vi "optionsAcq_channel_PD temperature mode.vi"(6 "read/write":enum16{"read", "write"}(ring), 8 "error in (no error)":errorcluster, 10 "PD sensitivity mode write":T1, 11 "OSAchannel in":refnum<class "OSAchannel.lvclass">) -> (0 "error out":errorcluster, 1 "channel.temp Variable":bool, 2 "PD sensitivity mode out":T1, 3 "OSAchannel out":refnum<class "OSAchannel.lvclass">, 5 "status FTSLib":i32)   [LabVIEW 2010, in "OSAchannel.lvclass"]
uses:
  OSAchannel.lvclass
  _misc/Thorlabs_FTS_misc.llb/PDTemperatureMode.ctl
  OSAchannel.lvclass/OSAchannel.ctl
  _dll/LVLib/FTSLib.lvlib
  OSA20X_misc.lvlib
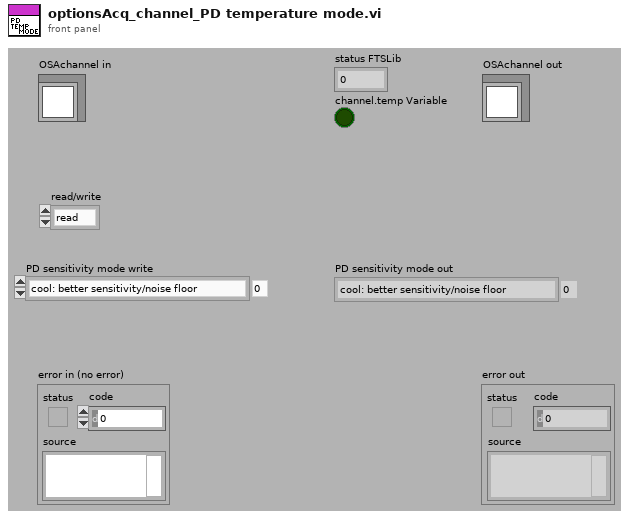
[diagram p1: front panel]
types:
  T1 = typedef "OSA20X_misc.lvlib/PDTemperatureMode.ctl" = enum16{"cool: better sensitivity/noise floor", "warm: extended wl range"}
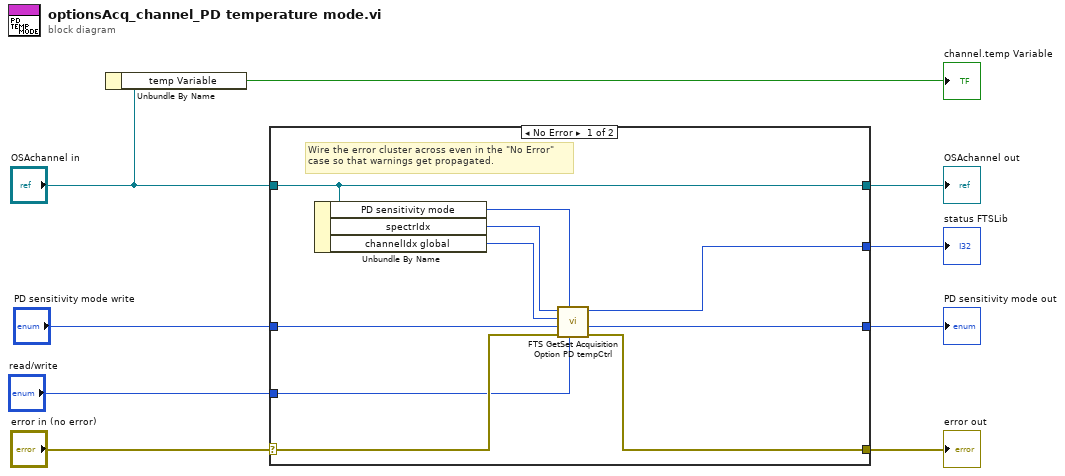
[diagram p0: block diagram]
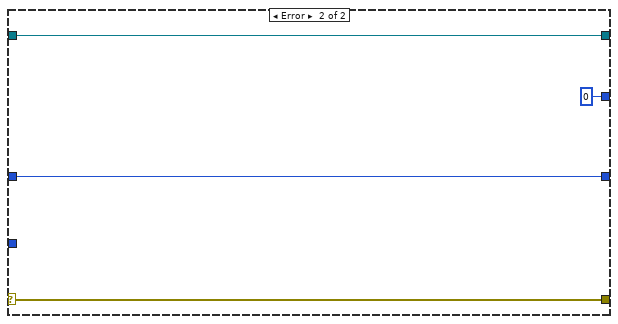
[diagram p2: hidden frame]
diagram:
  n1 = Unbundle By Name("OSAchannel in") -> ("temp Variable"=→"channel.temp Variable":bool)
  n2 = case shown="No Error" "error in (no error)" {
    selector: "error in (no error)" -> [w16 w23]
    tunnel: [w15 w23] -> w8
    tunnel: [w19 w22] -> w7
    tunnel: "OSAchannel in" -> [w19 w22]
    tunnel: "PD sensitivity mode write" -> [w14 w20]
    tunnel: "read/write" -> [w13 _]
    tunnel: [w11 w20] -> w4
    tunnel: [w10 0 ("status FTSLib")] -> w3
    frame No Error {
      # "Wire the error cluster across even in the \"No Error\"\ncase so that warnings get propagated."
      n3 = Unbundle By Name(w19) -> ("PD sensitivity mode"=w12:T1, "spectrIdx"=w18:u16, "channelIdx global"=w17:u16)
      n4 = call "FTS GetSet Acquisition Option PD tempCtrl.vi"("read/write"=w13, "PD sensitivity mode Pre"=w12, "error in"=w16, "PD sensitivity mode write"=w14, "channel index interferogram"=w17, "spectrometerIdx"=w18) -> ("error out"=w15:errorcluster, "PD sensitivity mode out"=w11:T1, "status FTSLib"=w10:i32)  [unwired: 3 in]
    }
    frame Error {
    }
  }
  "error out" <- w8
  "OSAchannel out" <- w7
  "PD sensitivity mode out" <- w4
  "status FTSLib" <- w3
